vi "Read Config.vi"(8 "error in (no error)":errorcluster) -> (0 "error out":errorcluster, 1 "STROKE PARAMETERS":dbl[](array[numeric]), 2 "ADC PARAMETERS":dbl[](array[numeric]), 3 "PID  PARAMETERS":dbl[](array[numeric]), 4 "CALIBRATION PARAMETERS":string[](array[string]), 5 "Stroke Calibration":string)   [LabVIEW 2025]
uses:
  Config file  FGV adv enum.ctl
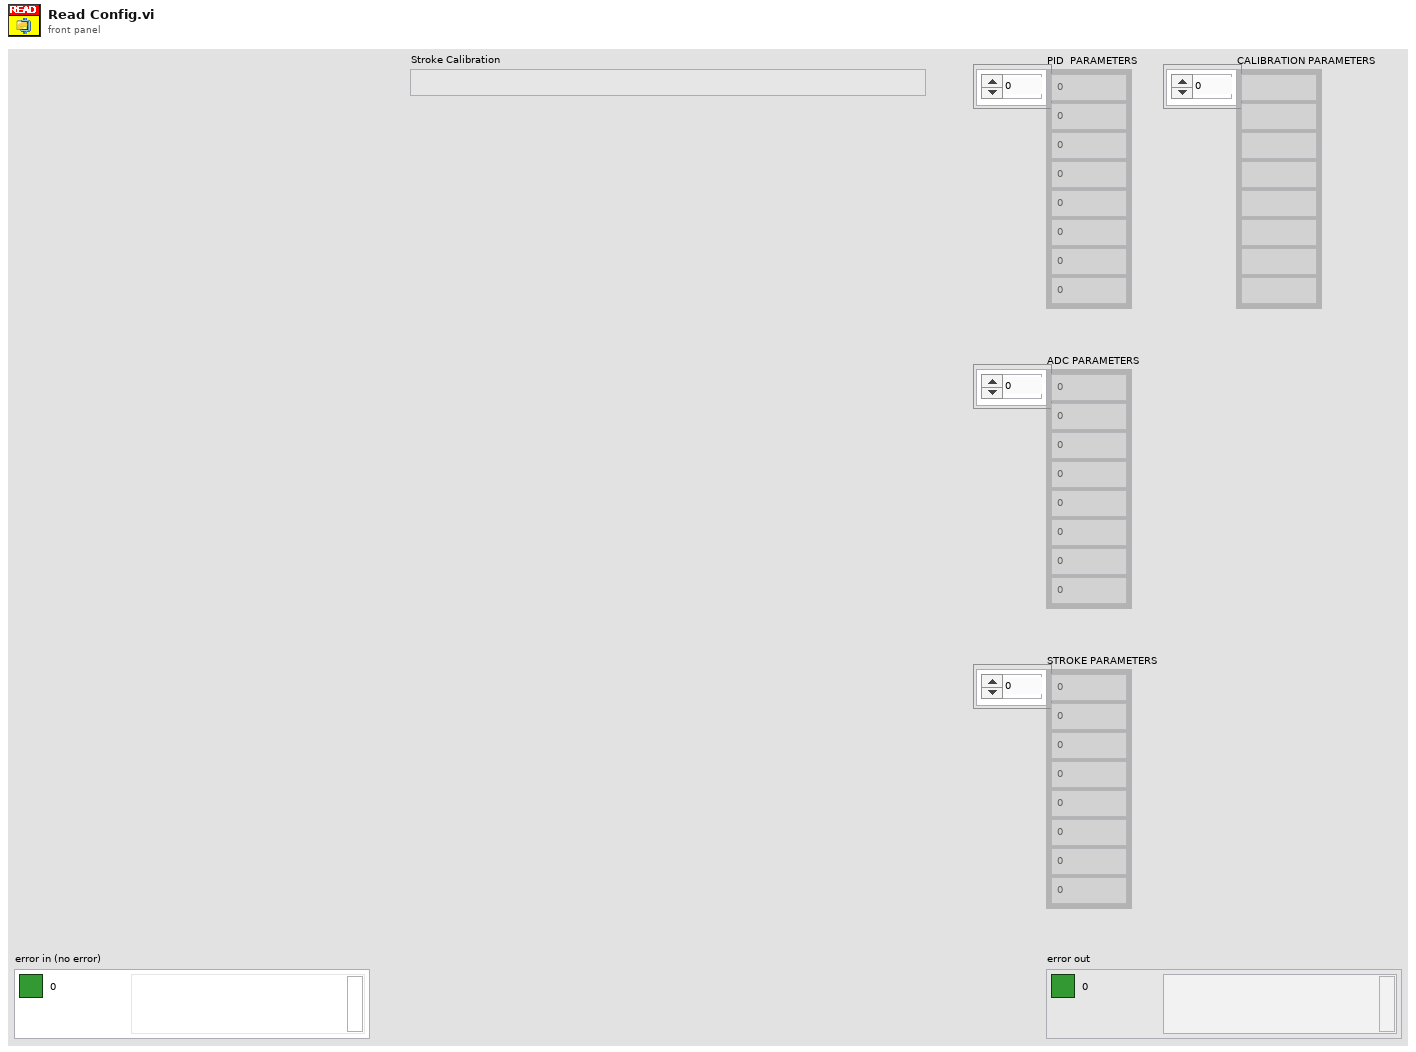
[diagram p1: front panel]
types:
  T1 = typedef "Config file  FGV adv enum.ctl" = enum16{"OPEN", "READ", "WRITE", "CLOSE"}
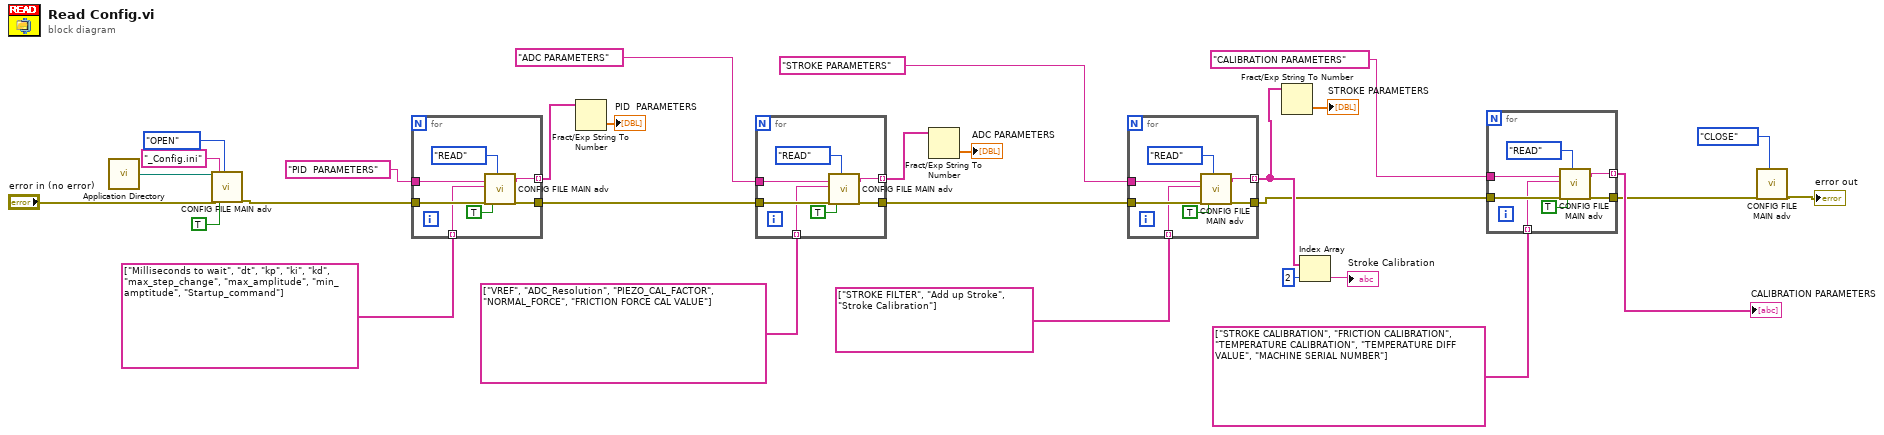
[diagram p0: block diagram]
diagram:
  n1 = call <vilib>:"Application Directory.vi"() -> ("Application Directory"=w17:path)
  n2 = call "CONFIG FILE MAIN adv.vi"("File Path"=w17, "error in"="error in (no error)", "file name"="_Config.ini", "PARAMETER/CONFIG"=TRUE, "Config Enum"=Config_file__FGV_adv_enum."OPEN") -> ("error out"=w16:errorcluster)  [unwired: 13 in, 1 out]
  n3 = for {
    tunnel: w16 -> [w35]
    tunnel: "PID  PARAMETERS" ("WRITE /READ SECTION") -> [w34]
    tunnel: string[] ["Milliseconds to wait", "dt", "kp", "ki", "kd", "max_step_change", "max_amplitude", "min_amptitude", "Startup_command"] -> [w33] mode=indexing
    tunnel: [w32] -> w12
    tunnel: [w31] -> w13 mode=indexing
    n4 = call "CONFIG FILE MAIN adv.vi"("WRITE /READ SECTION"=w34, "READ KEY"=w33, "error in"=w35, "PARAMETER/CONFIG"=TRUE, "Config Enum"=Config_file__FGV_adv_enum."READ") -> ("READ VALUE"=w31:string, "error out"=w32:errorcluster)  [unwired: 13 in]
  }
  n5 = Fract/Exp String To Number(string=w13) -> (number=→"PID  PARAMETERS":dbl[])  [unwired: 3 in, 1 out]
  n6 = for {
    tunnel: w12 -> [w42]
    tunnel: "ADC PARAMETERS" ("WRITE /READ SECTION") -> [w41]
    tunnel: [w40] -> w8
    tunnel: [w39] -> w9 mode=indexing
    tunnel: string[] ["VREF", "ADC_Resolution", "PIEZO_CAL_FACTOR", "NORMAL_FORCE", "FRICTION FORCE CAL VALUE"] -> [w37] mode=indexing
    n7 = call "CONFIG FILE MAIN adv.vi"("WRITE /READ SECTION"=w41, "READ KEY"=w37, "error in"=w42, "PARAMETER/CONFIG"=TRUE, "Config Enum"=Config_file__FGV_adv_enum."READ") -> ("READ VALUE"=w39:string, "error out"=w40:errorcluster)  [unwired: 13 in]
  }
  n8 = Fract/Exp String To Number(string=w9) -> (number=→"ADC PARAMETERS":dbl[])  [unwired: 3 in, 1 out]
  n9 = for {
    tunnel: w8 -> [w49]
    tunnel: "STROKE PARAMETERS" ("WRITE /READ SECTION") -> [w48]
    tunnel: [w47] -> w5
    tunnel: [w46] -> w21 mode=indexing
    tunnel: string[] ["STROKE FILTER", "Add up Stroke", "Stroke Calibration"] -> [w44] mode=indexing
    n10 = call "CONFIG FILE MAIN adv.vi"("WRITE /READ SECTION"=w48, "READ KEY"=w44, "error in"=w49, "PARAMETER/CONFIG"=TRUE, "Config Enum"=Config_file__FGV_adv_enum."READ") -> ("READ VALUE"=w46:string, "error out"=w47:errorcluster)  [unwired: 13 in]
  }
  n11 = Fract/Exp String To Number(string=w21) -> (number=→"STROKE PARAMETERS":dbl[])  [unwired: 3 in, 1 out]
  n12 = Index Array(array=w21, index=2) -> (element=→"Stroke Calibration":string)
  n13 = for {
    tunnel: w5 -> [w56]
    tunnel: "CALIBRATION PARAMETERS" ("WRITE /READ SECTION") -> [w55]
    tunnel: [w54] -> w1
    tunnel: [w53] -> w4 mode=indexing
    tunnel: string[] ["STROKE CALIBRATION", "FRICTION CALIBRATION", "TEMPERATURE CALIBRATION", "TEMPERATURE DIFF VALUE", "MACHINE SERIAL NUMBER"] -> [w51] mode=indexing
    n14 = call "CONFIG FILE MAIN adv.vi"("WRITE /READ SECTION"=w55, "READ KEY"=w51, "error in"=w56, "PARAMETER/CONFIG"=TRUE, "Config Enum"=Config_file__FGV_adv_enum."READ") -> ("READ VALUE"=w53:string, "error out"=w54:errorcluster)  [unwired: 13 in]
  }
  "CALIBRATION PARAMETERS" <- w4
  n15 = call "CONFIG FILE MAIN adv.vi"("error in"=w1, "Config Enum"=Config_file__FGV_adv_enum."CLOSE") -> ("error out"=→"error out":errorcluster)  [unwired: 16 in, 1 out]
